vi "TSM SSC DCPower Configure and Start Waveform Acquisition.vi"(0 "DCPower TSM in":T3, 5 "Sample Rate (Hz)":dbl=inf caption="Sample Rate (Max Hz)" format="%#_6p", 7 "Buffer Length (s)":dbl=1.0 caption="Buffer Length (1 second)" format="%#_6p", 11 "error in":errorcluster) -> (3 "Settings":T1 {"Previous Settings"."Triggers:Measure Trigger:Trigger Type" items=["Digital Edge"=1014, "Software Edge"=1015, "None"=1012]; "Previous Settings"."Measurement:Advanced:Measure When" items=["Automatically after Source Complete"=1025, "On Demand"=1026, "On Measure Trigger"=1027]; "Previous Settings"."Measurement:Aperture Time" format="%#_6p"; "Previous Settings"."Measurement:Aperture Time Units" items=["Seconds"=1028, "Power Line Cycles"=1029]}, 4 "DCPower TSM out":T3, 15 "error out":errorcluster)   [LabVIEW 2019]
doc: "This VI aborts the task, configures the tasks for waveform acquisition, initializes the task and starts the acquisition."
uses:
  TSM/TSM SSC DCPower.ctl
  <vilib>/NI_TestStand_SemiconductorModule/NI_TestStand_Semiconductor_Module.lvlibp/PinMap/PinQueryContext/MultiplePinMultipleSessionQueryContext/MultiplePinMultipleSessionQueryContext.lvclass
  SSC DCPower/SSC DCPower.ctl
  Shared SubVIs/TSM Pin Abstraction/TSM Pin Information.ctl
  Shared SubVIs/TSM Pin Abstraction/TSM Pin Type Identifier.ctl
  Shared SubVIs/TSM Pin Abstraction/TSM Expanded Pin Information.ctl
  SSC DCPower/Waveform Acquisition/SSC DCPower Waveform Acquisition Saved Settings.ctl
  SSC DCPower/Waveform Acquisition/SSC DCPower Waveform Acquisition Saved Setting.ctl
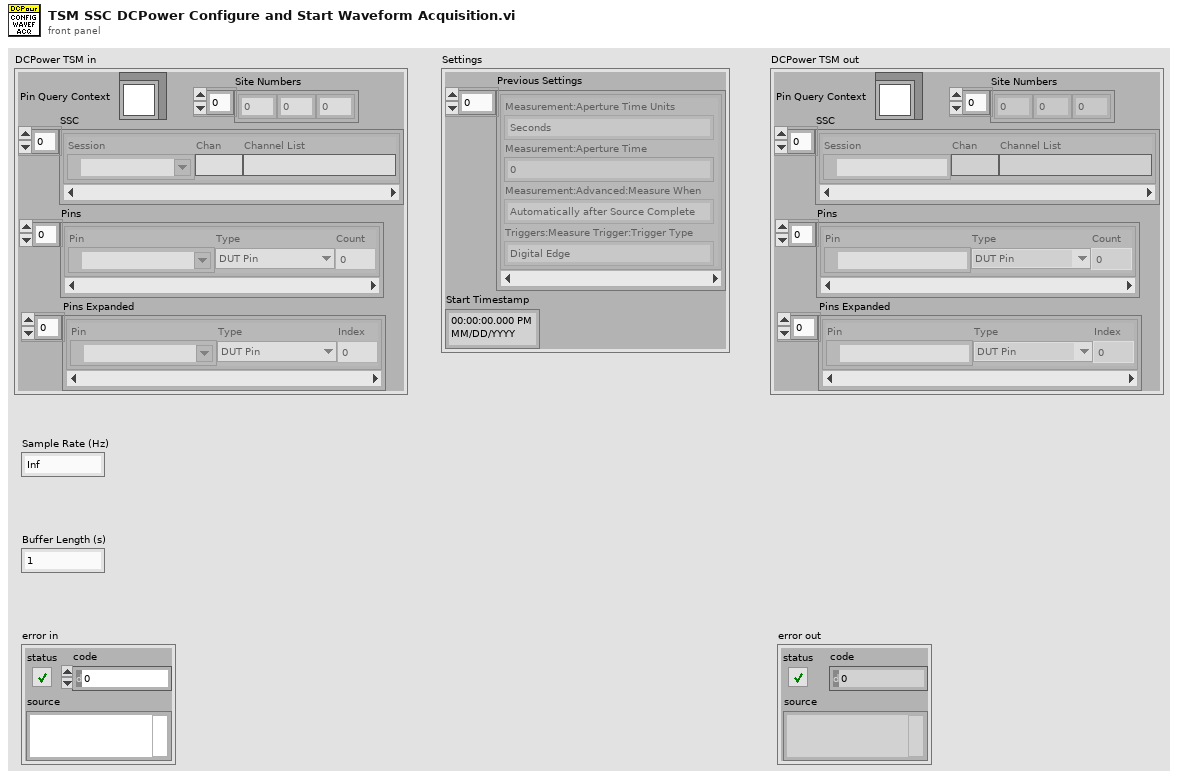
[diagram p1: front panel]
types:
  T1 = typedef "SSC DCPower Waveform Acquisition Saved Settings.ctl" = cluster{"Previous Settings":T2[], "Start Timestamp":timestamp}
  T2 = typedef "SSC DCPower Waveform Acquisition Saved Setting.ctl" = cluster{"Measurement:Aperture Time Units":i32, "Measurement:Aperture Time":dbl, "Measurement:Advanced:Measure When":i32, "Triggers:Measure Trigger:Trigger Type":i32}
  T3 = typedef "TSM SSC DCPower.ctl" = cluster{"Pin Query Context":refnum<class "MultiplePinMultipleSessionQueryContext.lvclass">, "SSC":T4[], "Site Numbers":i32[], "Pins":T5[], "Pins Expanded":T7[]}
  T4 = typedef "SSC DCPower.ctl" = cluster{"Session":refnum<k15>, "Chan":string, "Channel List":string}
  T5 = typedef "TSM Pin Information.ctl" = cluster{"Pin":tag, "Type":T6, "Count":i32}
  T6 = typedef "TSM Pin Type Identifier.ctl" = enum8{"DUT Pin", "System Pin", "Pin Group", "Not Determined"}
  T7 = typedef "TSM Expanded Pin Information.ctl" = cluster{"Pin":tag, "Type":T6, "Index":i32}
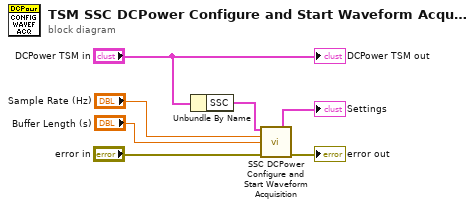
[diagram p0: block diagram]
diagram:
  n1 = Unbundle By Name("DCPower TSM in") -> ("SSC"=w1:T4[])
  n2 = call "SSC DCPower Configure and Start Waveform Acquisition.vi"("DCPower SSC in"=w1, "Sample Rate (Hz)"="Sample Rate (Hz)", "Buffer Length (s)"="Buffer Length (s)", "error in"="error in") -> ("Settings"=→"Settings":T1, "error out"=→"error out":errorcluster)  [unwired: 9 in, 1 out]
  "DCPower TSM out" <- "DCPower TSM in"
